vi "Load_Geometry_ColDet.vi"(8 "error in":errorcluster, 9 "Probe Path Array":path[](array[path]), 10 "Moving Path Array":path[](array[path]), 11 "Static Path Array":path[](array[path])) -> (0 "error out":errorcluster, 1 "Number Moving":i32, 2 "Number Static":i32)   [LabVIEW 2011]
doc: "This VI is used to load in the relevant geometry for the tunnel model. The various models (and only those models!) should be read in from seperate folders. The probe folder should contain only the probe gemotery, a single .3DS file. The Static geometry is stationary and cannot be moved. The Moving geometry is movable through rotations and translations. .3DS files can be created in 3DS Max, a downloadable software that is free to students. Goto the autodesk website to download."
uses:
  Enflo_Collision_Detection.dll
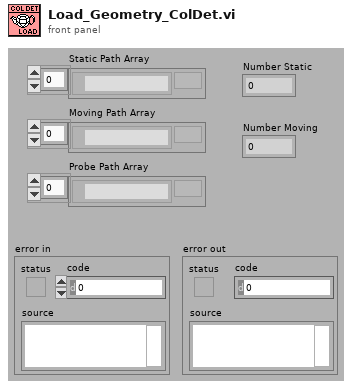
[diagram p1: front panel]
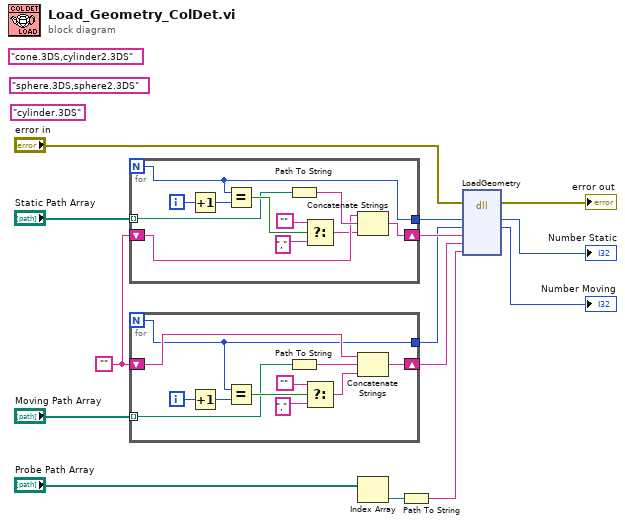
[diagram p0: block diagram]
diagram:
  w3 = ""
  (unwired) "sphere.3DS,sphere2.3DS" ("Moving Files")
  (unwired) "cone.3DS,cylinder2.3DS" ("Static Files")
  (unwired) "cylinder.3DS" ("Static Files")
  n1 = for {
    N -> [w15]
    tunnel: "Static Path Array" -> [w16] mode=indexing
    shift-right: [w23] -> w10
    shift-left: w3 -> [w24]
    tunnel: [w15] -> w7
    i -> [w22]
    n2 = Increment(x=w22) -> (x+1=w17:i32)
    n3 = Equal?(x=w15, y=w17) -> (x = y?=w21:bool)
    n4 = Path To String(path=w16) -> (string=w25:string)
    n5 = Select(t="", s=w21, f="," ("string")) -> (s? t:f=w19:string)
    n6 = Concatenate Strings(w24, w25, w19) -> (w23:string)
  }
  n7 = for {
    N -> [w26]
    tunnel: "Moving Path Array" -> [w27] mode=indexing
    shift-right: [w34] -> w2
    shift-left: w3 -> [w35]
    tunnel: [w26] -> w1
    i -> [w33]
    n8 = Increment(x=w33) -> (x+1=w28:i32)
    n9 = Equal?(x=w26, y=w28) -> (x = y?=w32:bool)
    n10 = Path To String(path=w27) -> (string=w36:string)
    n11 = Select(t="", s=w32, f="," ("string")) -> (s? t:f=w30:string)
    n12 = Concatenate Strings(w35, w36, w30) -> (w34:string)
  }
  n13 = Index Array(array="Probe Path Array") -> (element=w4:path)  [unwired: 1 in]
  n14 = Path To String(path=w4) -> (string=w9:string)
  n15 = dll-call lib="C:/Enflo_Software_SVN/EnFloSW/Anemometry/Anemometry Sub Vis/Collision_Detection/Enflo_Collision_Detection.dll" fn="LoadGeometry"(error in="error in", "Number Static"=w7, "Number Moving"=w1, "Static Files"=w10, "Moving Files"=w2, "Probe File"=w9) -> (error out=→"error out":errorcluster, "Number Static"=→"Number Static":i32, "Number Moving"=→"Number Moving":i32)  [unwired: 6 in, 1 out]
